vi "BCtr_Enable.vi"(7 "error in (no error)":errorcluster, 9 "Enable":bool, 10 "CtrCfg":T1 {"BaseAddrOut" format="%x"}) -> (0 "error out":errorcluster, 2 "Ack":bool, 3 "CtrCfg":T1 {"BaseAddrOut" format="%x"})   [LabVIEW 2016]
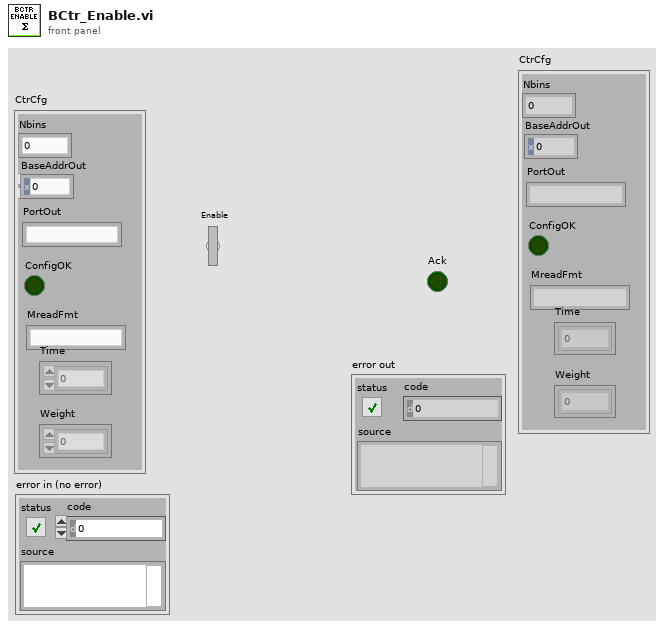
[diagram p1: front panel]
types:
  T1 = cluster{"Nbins":u16, "BaseAddrOut":u16, "PortOut":string, "ConfigOK":bool, "MreadFmt":string, "Time":dbl[], "Weight":dbl[]}
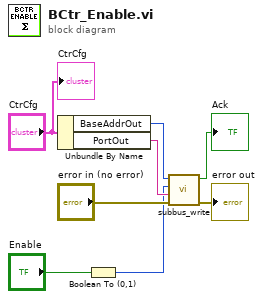
[diagram p0: block diagram]
diagram:
  n1 = Unbundle By Name("CtrCfg") -> ("BaseAddrOut"=w7:u16, "PortOut"=w8:string)
  n2 = Boolean To (0,1)(Boolean="Enable") -> (0, 1=w2:i16)
  n3 = call "subbus_write.vi"("error in (no error)"="error in (no error)", "PortIn"=w8, "Data"=w2, "Address"=w7) -> ("error out"=→"error out":errorcluster, "Ack"=→"Ack":bool)  [unwired: 5 in, 1 out]
  "CtrCfg" <- "CtrCfg"
